vi "LKIF2_DataStorageGetStatus.vi"(8 "error in (no error)":errorcluster {"code" format="%x"}) -> (0 "error out":errorcluster {"code" format="%x"}, 2 "NumStorageData":i32, 3 "IsStorage":bool)   [LabVIEW 2013, in "Keyence LK-G5000.lvlib"]
uses:
  <instrlib>/Keyence LK-G5000/Keyence LK-G5000.lvlib
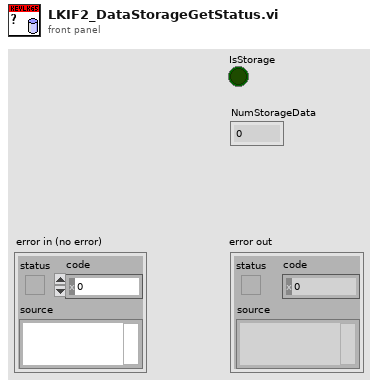
[diagram p1: front panel]
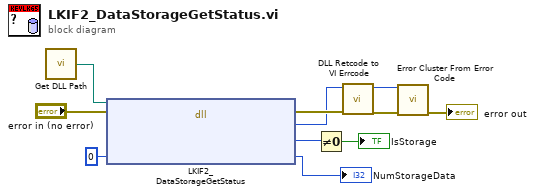
[diagram p0: block diagram]
diagram:
  n1 = call <instrlib>:"Get DLL Path.vi"() -> ("DLL Path"=w2:path)  [unwired: 1 in]
  n2 = dll-call lib="C:/Program Files/National Instruments/LabVIEW 2011/instr.lib/Keyence LK-G5000/LKIF2.dll" fn="LKIF2_DataStorageGetStatus"(path in=w2, error in="error in (no error)", "NumStorageData"=0) -> (error out=w7:errorcluster, "RC"=w6:i32, "IsStorage"=w5:i32, "NumStorageData"=→"NumStorageData":i32)  [unwired: 2 in, 1 out]
  n3 = Not Equal To 0?(x=w5) -> (x != 0?=→"IsStorage":bool)
  n4 = call <instrlib>:"DLL Retcode to VI Errcode.vi"("error in (no error)"=w7, "DLL Retcode"=w6) -> ("error out"=w11:errorcluster, "VI Errcode"=w10:i32)  [unwired: 8 in]
  n5 = call <vilib>:"Error Cluster From Error Code.vi"("error in (no error)"=w11, "error code (0)"=w10) -> ("error out"=→"error out":errorcluster)  [unwired: 7 in]
